vi "pwm test.vi"() -> ()   [LabVIEW 2015]
panel:
  in  "number of samples":i32=10000
  in  "rate":dbl=100000.0
  out "data":dynamicdata(graph)
  in  "Duty Cycle (%)":dbl=50.0 format="%_4g"
  out "Square":dynamicdata(graph)
  in  "stop":bool
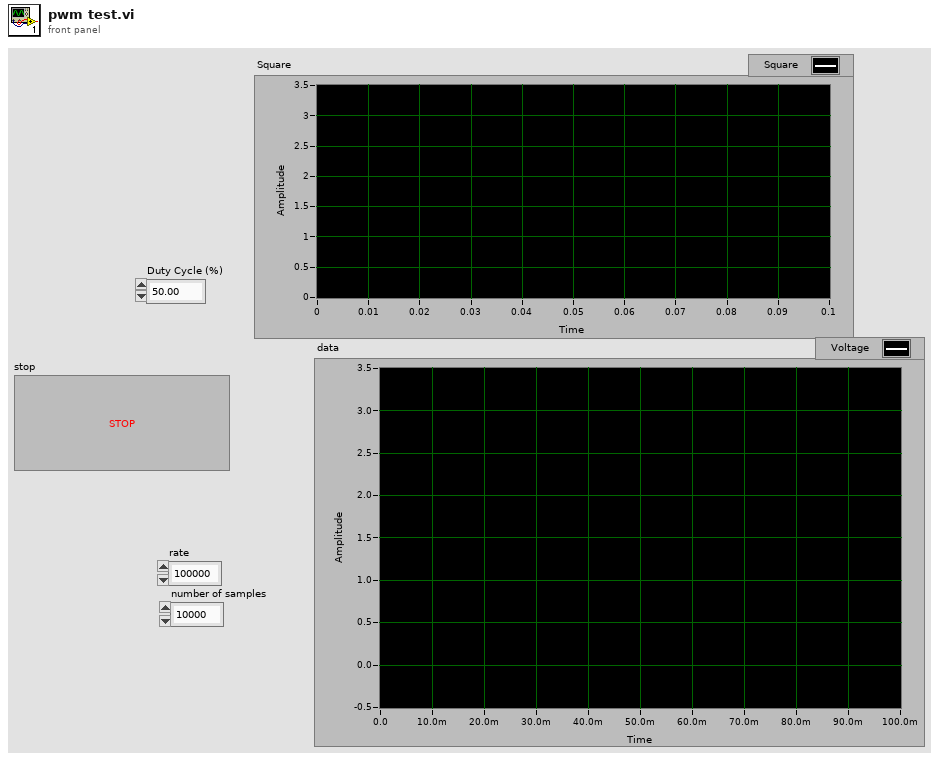
[diagram p1: front panel]
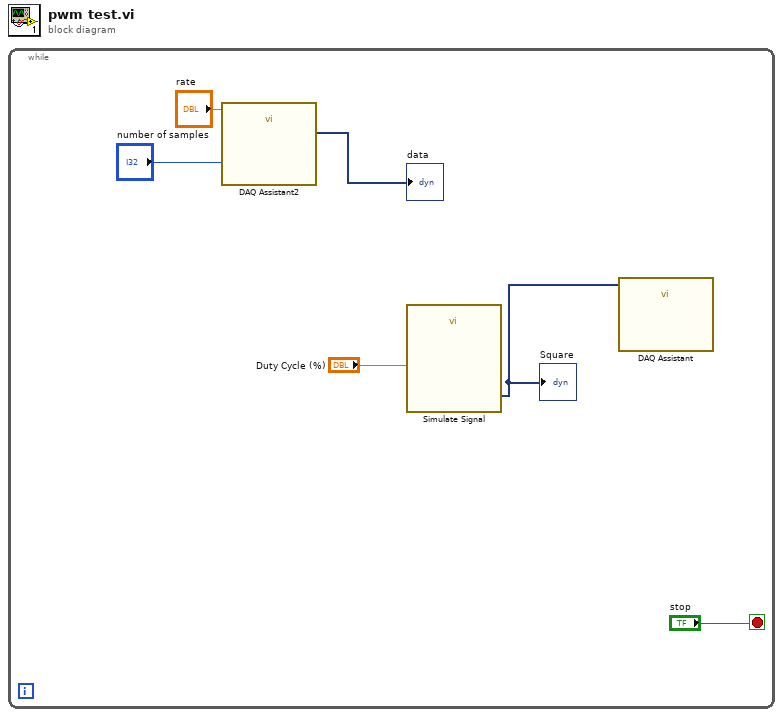
[diagram p0: block diagram]
diagram:
  n1 = while {
    stop <- "stop" stop-if-true
    n2 = call "DAQ Assistant2"("rate"="rate", "number of samples"="number of samples") -> ("data"=→"data":dynamicdata)  [unwired: 15 in, 2 out]
    n3 = call "Simulate Signal"("Duty Cycle (%)"="Duty Cycle (%)") -> ("Square"=w6:dynamicdata)  [unwired: 13 in, 1 out]
    "Square" <- w6
    n4 = call "DAQ Assistant"("data"=w6) -> ()  [unwired: 16 in, 3 out]
  }
